vi "Matrix Balance.vi"   [LabVIEW 2020, in "NI_AALPro.lvlib"]
doc: "Balances the general matrix <B>Input Matrix</B> to improve the accuracy of computed eigenvalues and eigenvectors. Wire data to the <B>Input Matrix</B> input to determine the polymorphic instance to use or manually select the instance."
uses:
  NI_AALPro.lvlib
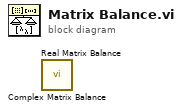
[diagram p0: block diagram]
diagram:
  n1 = call "Complex Matrix Balance.vi"() -> ()  [unwired: 7 in, 5 out]
  n2 = call "Real Matrix Balance.vi"() -> ()  [unwired: 7 in, 5 out]
